vi "NI9623_SUB-VI_Array1sizeAdapter.vi"(8 "error in (no error)":errorcluster, 11 "Channel Values":variant) -> (3 "Real 2D Array":dbl[][](array[numeric]))   [LabVIEW 2020]
uses:
  <vilib>/Analysis/Matrix/Numeric/Conversions/Array To Matrix - RA.vi
  <vilib>/Analysis/Matrix/Numeric/Conversions/Matrix To Array - RM.vi
  <vilib>/Analysis/Matrix/NI_Matrix.lvlib
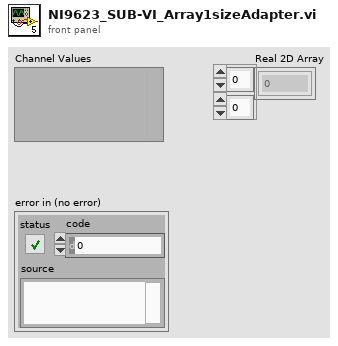
[diagram p1: front panel]
types:
  T1 = typedef "NI_Matrix.lvlib/RealMatrix.ctl" = dbl[][]
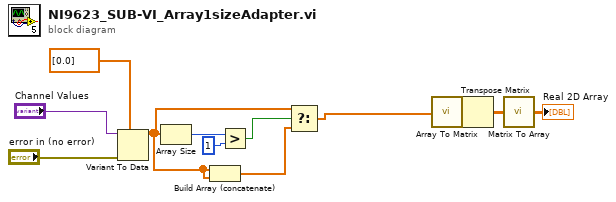
[diagram p0: block diagram]
diagram:
  n1 = Variant To Data(error in="error in (no error)", type=dbl[] [0.0] ("Channel Values Array"), Variant="Channel Values") -> (data=w3:dbl[])  [unwired: 1 out]
  n2 = Array Size(array=w3) -> (size(s)=w10:i32)
  n3 = Build Array (concatenate)(w3, w3) -> (w2:dbl[])
  n4 = Greater?(x=w10, y=1) -> (0:w12:bool)
  n5 = Select(t=w3, s=w12, f=w2) -> (s? t:f=w1:dbl[])
  n6 = call-poly <vilib>:"Array To Matrix.vi"("Real 1D Array"=w1) -> ("Real Matrix (Column Vector)"=w7:T1)
  n7 = Transpose Matrix(1:w7) -> (0:w8:T1)
  n8 = call-poly <vilib>:"Matrix To Array.vi"("Real Matrix"=w8) -> ("Real 2D Array"=→"Real 2D Array":dbl[][])
